vi "Query Output.vi"(8 "error in (no error)":errorcluster, 10 "Channel (0: Channel 1)":T1 items=["Channel 1", "Channel 2"], 11 "VISA resource name":refnum<visa-resource-name>) -> (0 "error out":errorcluster, 2 "Output Enabled?":bool=TRUE, 3 "VISA resource name out":refnum<visa-resource-name>)   [LabVIEW 2015, in "Tektronix AFG 3000 Series.lvlib"]
uses:
  Tektronix AFG 3000 Series.lvlib
  controls.llb/Channel.ctl
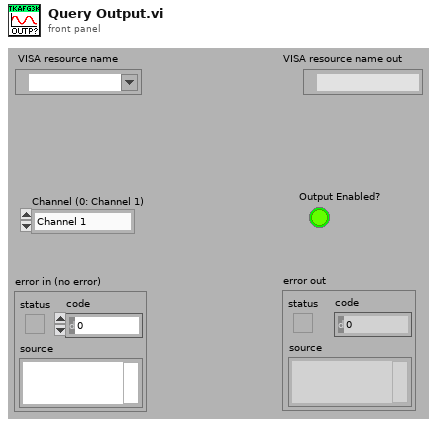
[diagram p1: front panel]
types:
  T1 = typedef "Channel.ctl" = u16
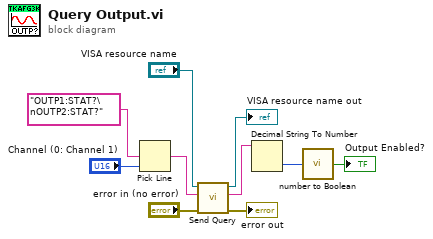
[diagram p0: block diagram]
diagram:
  n1 = Pick Line(multi-line string="OUTP1:STAT?\nOUTP2:STAT?" ("string (\"\")"), line index="Channel (0: Channel 1)") -> (output string=w8:string)  [unwired: 1 out]
  n2 = call "Send Query.vi"("error in (no error)"="error in (no error)", "write buffer"=w8, "VISA resource name"="VISA resource name") -> ("error out"=→"error out":errorcluster, "read buffer"=w2:string, "VISA resource name out"=→"VISA resource name out":refnum<visa-resource-name>)  [unwired: 1 in, 5 out]
  n3 = Decimal String To Number(string=w2) -> (number=w1:i32)  [unwired: 3 out]
  n4 = call "number to Boolean.vi"("Numeric"=w1) -> ("Boolean"=→"Output Enabled?":bool)
